vi "Save Image by User.vi"(8 "error in (no error)":errorcluster, 11 "HIJ Vision Application in":refnum<class "HIJ Vision Application.lvclass">) -> (0 "error out":errorcluster, 3 "HIJ Vision Application out":refnum<class "HIJ Vision Application.lvclass">)   [LabVIEW 2020, in "HIJ Vision Application.lvlib" / "HIJ Vision Application.lvclass"]
uses:
  HIJ Vision Application.lvclass
  HIJ Vision Application.lvclass/HIJ Vision Application.ctl
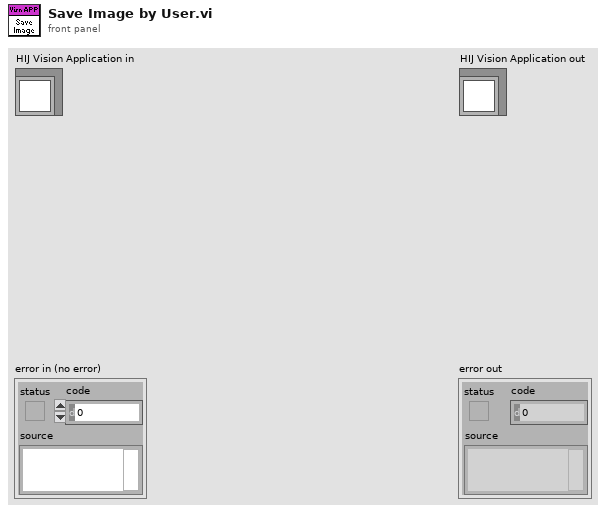
[diagram p1: front panel]
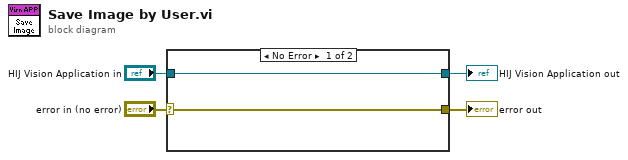
[diagram p0: block diagram]
diagram:
  n1 = case shown="No Error" "error in (no error)" {
    selector: "error in (no error)" -> [w5 w8]
    tunnel: [w5 w8] -> w3
    tunnel: [w6 w7] -> w1
    tunnel: "HIJ Vision Application in" -> [w6 w7]
    frame No Error {
    }
    frame Error {
    }
  }
  "error out" <- w3
  "HIJ Vision Application out" <- w1
